vi "Day 5 - Supply Stacks.vi"() -> ()   [LabVIEW 2020, in "AoC 2022.lvlib"]
uses:
  AoC 2022.lvlib
panel:
  out "Puzzle Part-2 Answer":string
  out "Puzzle Answer":string
  in  "Puzzle Input":string="    [D]    \n[N] [C]    \n[Z] [M] [P]\n 1   2   3 \n\nmove 1 from 2 to 1\nmove 3 from 1 to 3\nmove 2 from 2 to 1\nmove 1 from 1 to 2"
  # "Press Ctrl+M & Enter the Puzzle Input and run the VI"
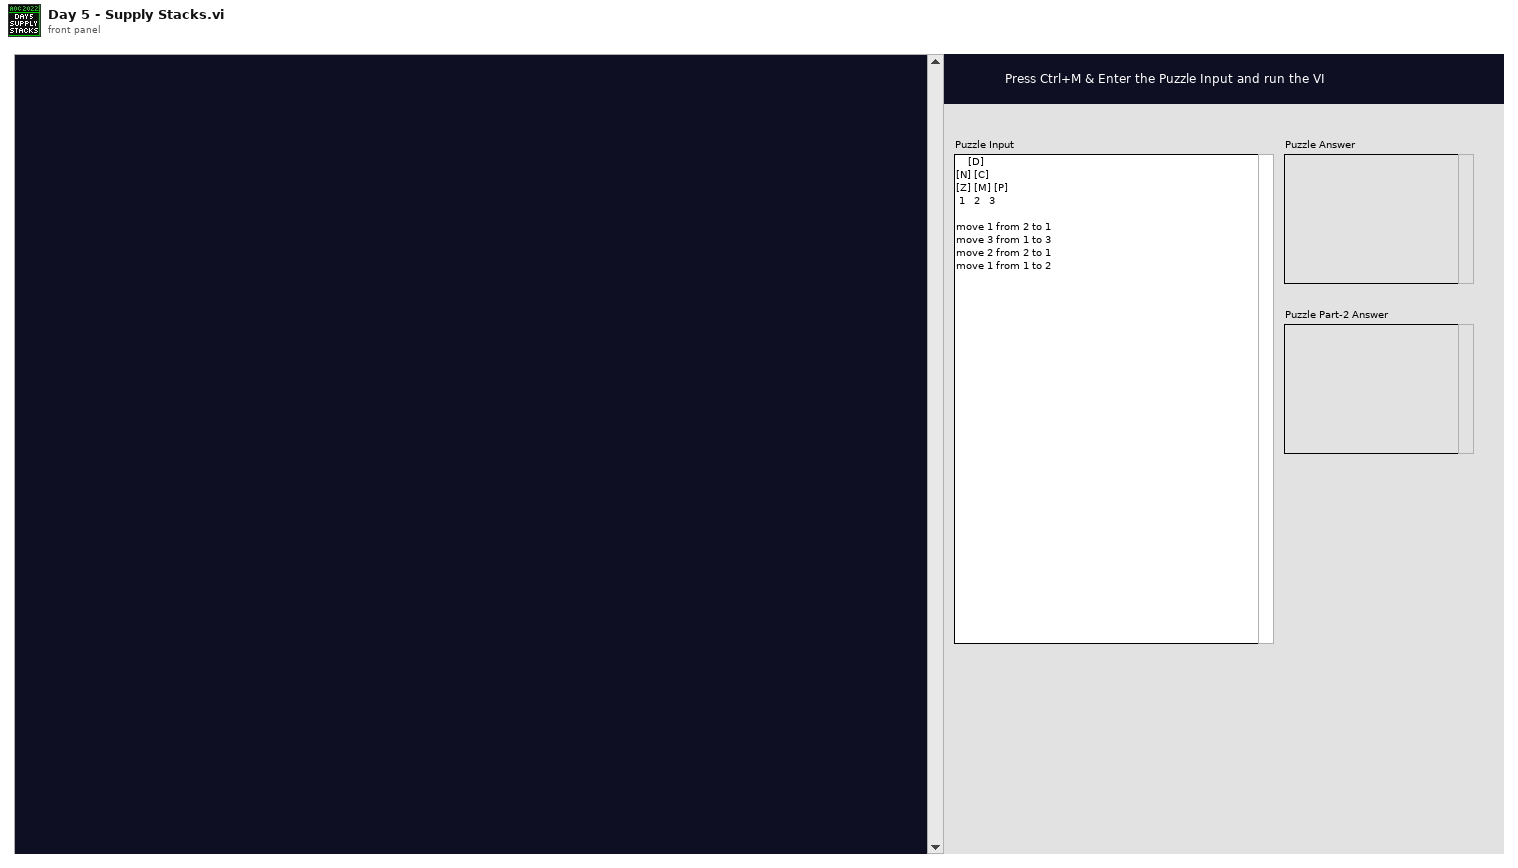
[diagram p1: front panel]
types:
  T1 = typedef "AoC 2022.lvlib/Cargo.ctl" = map{i32, string[]}
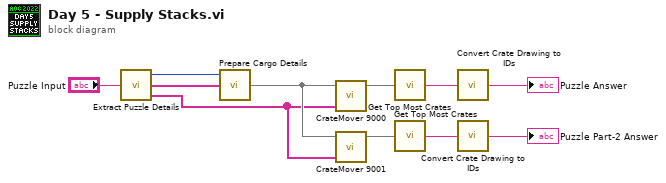
[diagram p0: block diagram]
diagram:
  n1 = call "Extract Puzzle Details.vi"("Puzzle Input"="Puzzle Input") -> ("#Stacks"=w9:i32, "Stacks Drawing"=w10:string[], "Crane Operator Instructions"=w2:string[])
  n2 = call "Prepare Cargo Details.vi"("Stacks Drawing"=w10, "#Stacks"=w9) -> ("Cargo"=w3:T1)  [unwired: 1 in]
  n3 = call "CrateMover 9000.vi"("Crane Instructions"=w2, "Cargo in"=w3) -> ("Cargo out"=w4:T1)  [unwired: 3 in]
  n4 = call "CrateMover 9001.vi"("Crane Instructions"=w2, "Cargo in"=w3) -> ("Cargo out"=w1:T1)  [unwired: 3 in]
  n5 = call "Get Top Most Crates.vi"("Cargo"=w4) -> ("Top Most Crates"=w8:string)
  n6 = call "Get Top Most Crates.vi"("Cargo"=w1) -> ("Top Most Crates"=w5:string)
  n7 = call "Convert Crate Drawing to IDs.vi"("Crate Drawing"=w8) -> ("Crate IDs"=→"Puzzle Answer":string)
  n8 = call "Convert Crate Drawing to IDs.vi"("Crate Drawing"=w5) -> ("Crate IDs"=→"Puzzle Part-2 Answer":string)
